vi "Standard_Channel_Names.vi"() -> (0 "Standard Ch Names":string[](array[string])=["X Ch Name", "Y Ch Name", "Z Ch Name", "Wind Direction", "Coord System", "STL Filename", "U Ch Name", "V Ch Name", "W Ch Name"])   [LabVIEW 2022 SP3]
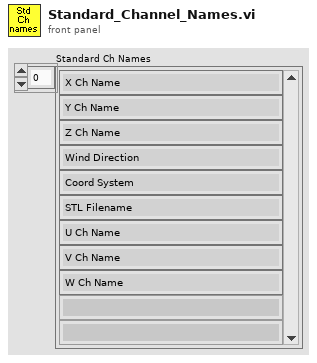
[diagram p1: front panel]
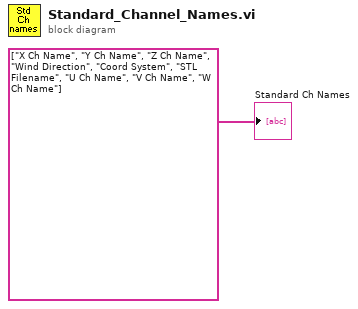
[diagram p0: block diagram]
diagram:
  "Standard Ch Names" <- string[] ["X Ch Name", "Y Ch Name", "Z Ch Name", "Wind Direction", "Coord System", "STL Filename", "U Ch Name", "V Ch Name", "W Ch Name"] ("1D Info Out")
